vi "Zadanie3.vi"() -> ()   [LabVIEW 2011]
panel:
  in  "Пауза":dbl
  out "Число 2":dbl
  out "Число 1":dbl
  out "График суммы":dbl(graph)
  out "Сумма":dbl
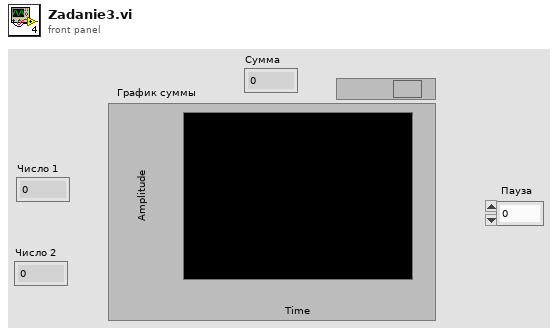
[diagram p1: front panel]
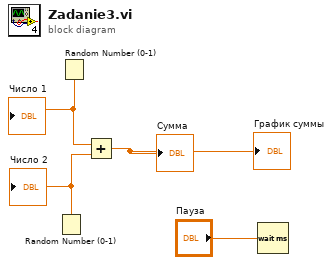
[diagram p0: block diagram]
diagram:
  n1 = Random Number (0-1)() -> (number: 0 to 1=w3:dbl)
  "Число 2" <- w3
  n2 = Random Number (0-1)() -> (number: 0 to 1=w2:dbl)
  "Число 1" <- w2
  n3 = Add(x=w2, y=w3) -> (x+y=→"Сумма" →"График суммы":dbl)
  n4 = Wait (ms)(milliseconds to wait="Пауза") -> ()  [unwired: 1 out]
